vi "myRIO_BRig_Host_formatData_getHeaders_dataLC.vi"() -> (3 "output_stringArray_dataLC":string[](array[string]))   [LabVIEW 2014]
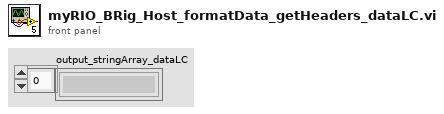
[diagram p1: front panel]
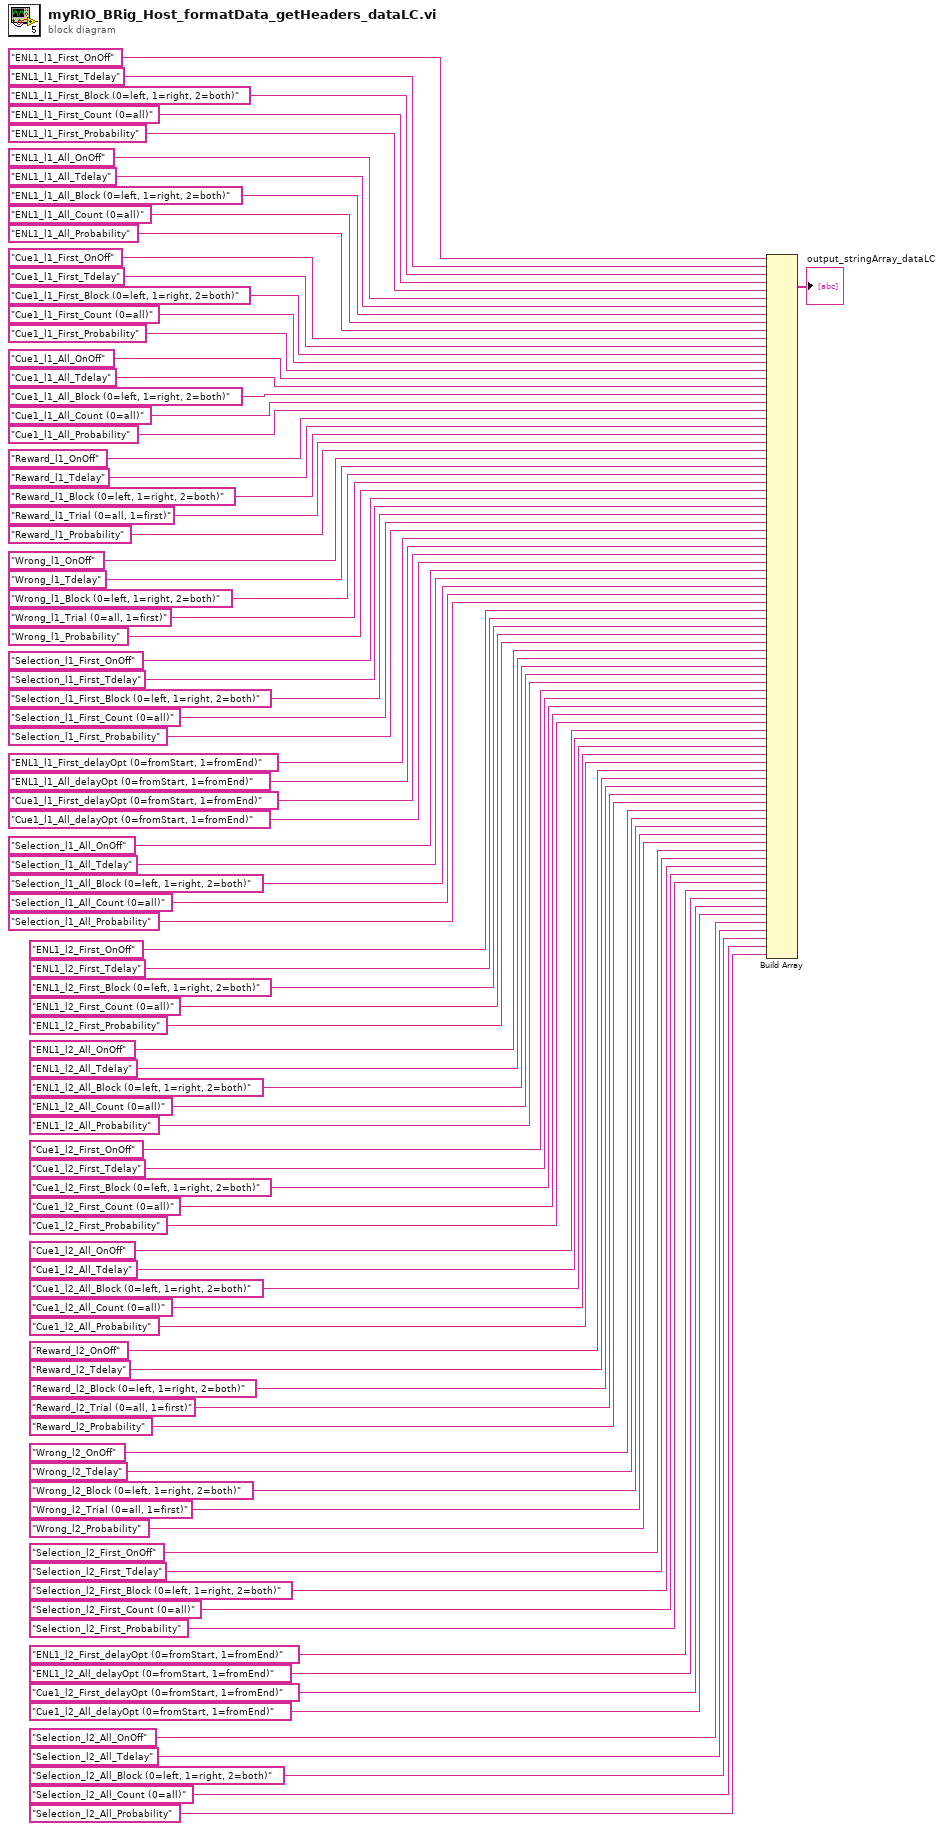
[diagram p0: block diagram]
diagram:
  n1 = Build Array("ENL1_l1_First_OnOff", "ENL1_l1_First_Tdelay", "ENL1_l1_First_Block (0=left, 1=right, 2=both)", "ENL1_l1_First_Count (0=all)", "ENL1_l1_First_Probability", "ENL1_l1_All_OnOff", "ENL1_l1_All_Tdelay", "ENL1_l1_All_Block (0=left, 1=right, 2=both)", "ENL1_l1_All_Count (0=all)", "ENL1_l1_All_Probability", "Cue1_l1_First_OnOff", "Cue1_l1_First_Tdelay", "Cue1_l1_First_Block (0=left, 1=right, 2=both)", "Cue1_l1_First_Count (0=all)", "Cue1_l1_First_Probability", "Cue1_l1_All_OnOff", "Cue1_l1_All_Tdelay", "Cue1_l1_All_Block (0=left, 1=right, 2=both)", "Cue1_l1_All_Count (0=all)", "Cue1_l1_All_Probability", "Reward_l1_OnOff", "Reward_l1_Tdelay", "Reward_l1_Block (0=left, 1=right, 2=both)", "Reward_l1_Trial (0=all, 1=first)", "Reward_l1_Probability", "Wrong_l1_OnOff", "Wrong_l1_Tdelay", "Wrong_l1_Block (0=left, 1=right, 2=both)", "Wrong_l1_Trial (0=all, 1=first)", "Wrong_l1_Probability", "Selection_l1_First_OnOff", "Selection_l1_First_Tdelay", "Selection_l1_First_Block (0=left, 1=right, 2=both)", "Selection_l1_First_Count (0=all)", "Selection_l1_First_Probability", "ENL1_l1_First_delayOpt (0=fromStart, 1=fromEnd)", "ENL1_l1_All_delayOpt (0=fromStart, 1=fromEnd)", "Cue1_l1_First_delayOpt (0=fromStart, 1=fromEnd)", "Cue1_l1_All_delayOpt (0=fromStart, 1=fromEnd)", "Selection_l1_All_OnOff", "Selection_l1_All_Tdelay", "Selection_l1_All_Block (0=left, 1=right, 2=both)", "Selection_l1_All_Count (0=all)", "Selection_l1_All_Probability", "ENL1_l2_First_OnOff", "ENL1_l2_First_Tdelay", "ENL1_l2_First_Block (0=left, 1=right, 2=both)", "ENL1_l2_First_Count (0=all)", "ENL1_l2_First_Probability", "ENL1_l2_All_OnOff", "ENL1_l2_All_Tdelay", "ENL1_l2_All_Block (0=left, 1=right, 2=both)", "ENL1_l2_All_Count (0=all)", "ENL1_l2_All_Probability", "Cue1_l2_First_OnOff", "Cue1_l2_First_Tdelay", "Cue1_l2_First_Block (0=left, 1=right, 2=both)", "Cue1_l2_First_Count (0=all)", "Cue1_l2_First_Probability", "Cue1_l2_All_OnOff", "Cue1_l2_All_Tdelay", "Cue1_l2_All_Block (0=left, 1=right, 2=both)", "Cue1_l2_All_Count (0=all)", "Cue1_l2_All_Probability", "Reward_l2_OnOff", "Reward_l2_Tdelay", "Reward_l2_Block (0=left, 1=right, 2=both)", "Reward_l2_Trial (0=all, 1=first)", "Reward_l2_Probability", "Wrong_l2_OnOff", "Wrong_l2_Tdelay", "Wrong_l2_Block (0=left, 1=right, 2=both)", "Wrong_l2_Trial (0=all, 1=first)", "Wrong_l2_Probability", "Selection_l2_First_OnOff", "Selection_l2_First_Tdelay", "Selection_l2_First_Block (0=left, 1=right, 2=both)", "Selection_l2_First_Count (0=all)", "Selection_l2_First_Probability", "ENL1_l2_First_delayOpt (0=fromStart, 1=fromEnd)", "ENL1_l2_All_delayOpt (0=fromStart, 1=fromEnd)", "Cue1_l2_First_delayOpt (0=fromStart, 1=fromEnd)", "Cue1_l2_All_delayOpt (0=fromStart, 1=fromEnd)", "Selection_l2_All_OnOff", "Selection_l2_All_Tdelay", "Selection_l2_All_Block (0=left, 1=right, 2=both)", "Selection_l2_All_Count (0=all)", "Selection_l2_All_Probability") -> (→"output_stringArray_dataLC":string[])
